vi "readAnPinVal.vi"(3 "YLDRMErrorInp":errorcluster, 4 "pin":u8, 5 "YLDRMPortInp":refnum<visa-resource-name>) -> (0 "YLDRMErrorOut":errorcluster, 1 "out":u16, 2 "YLDRMPortOut":refnum<visa-resource-name>)   [LabVIEW 2015]
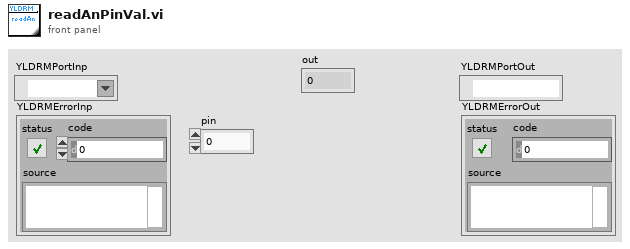
[diagram p1: front panel]
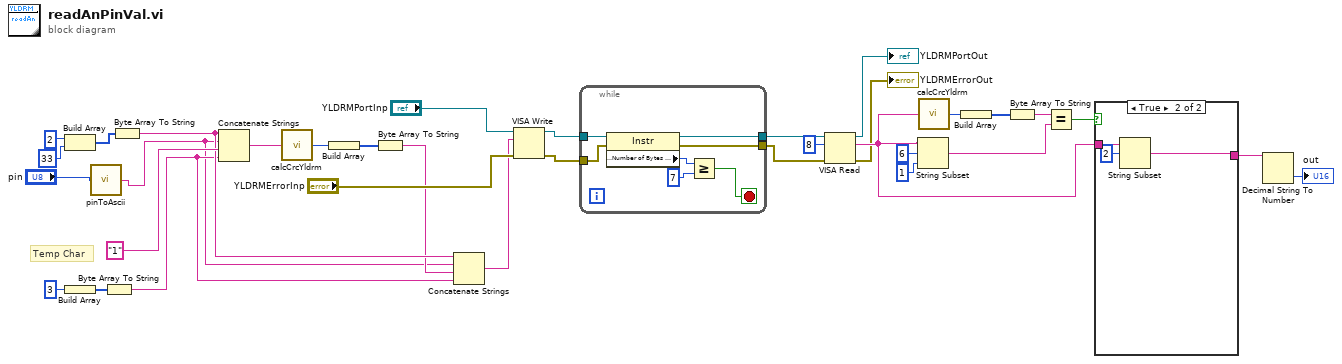
[diagram p0: block diagram]
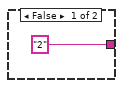
[diagram p2: hidden frame]
diagram:
  # "Temp Char"
  n1 = Build Array(2, 33) -> (w32:i32[])
  n2 = Build Array(3) -> (w30:i32[])
  n3 = call "pinToAscii.vi"("inp"="pin") -> ("out"=w1:string)
  n4 = Byte Array To String(unsigned byte array=w30) -> (string=w6:string)
  n5 = Byte Array To String(unsigned byte array=w32) -> (string=w8:string)
  n6 = Concatenate Strings(w8, w1, "1", w6) -> (w27:string)
  n7 = call "calcCrcYldrm.vi"("inpStr"=w27) -> ("crcVal"=w29:u8)
  n8 = Build Array(w29) -> (w28:u8[])
  n9 = Byte Array To String(unsigned byte array=w28) -> (string=w7:string)
  n10 = Concatenate Strings(w8, w1, w7, w6) -> (w5:string)
  n11 = VISA Write(VISA resource name="YLDRMPortInp", write buffer=w5, error in (no error)="YLDRMErrorInp") -> (VISA resource name out=w23:refnum<visa-resource-name>, error out=w22:errorcluster)  [unwired: 1 out]
  n12 = while {
    tunnel: w23 -> [w41]
    tunnel: w22 -> [w40]
    tunnel: [w39] -> w21
    tunnel: [w38] -> w20
    stop <- w35 stop-if-true
    n13 = property class="Instr"(reference=w41, error in=w40) -> (reference out=w39:refnum<visa-resource-name>, error out=w38:errorcluster, "Serial Settings:Number of Bytes at Serial Port"=w37:u32)
    n14 = Greater Or Equal?(x=w37, y=u32 7) -> (x >= y?=w35:bool)
  }
  n15 = VISA Read(VISA resource name=w21, byte count=u32 8, error in (no error)=w20) -> (VISA resource name out=→"YLDRMPortOut":refnum<visa-resource-name>, read buffer=w11:string, error out=→"YLDRMErrorOut":errorcluster)  [unwired: 1 out]
  n16 = String Subset(string=w11, offset (0)=6, length (rest)=1 ("length (rest)")) -> (substring=w13:string)
  n17 = call "calcCrcYldrm.vi"("inpStr"=w11) -> ("crcVal"=w17:u8)
  n18 = Build Array(w17) -> (w18:u8[])
  n19 = Byte Array To String(unsigned byte array=w18) -> (string=w14:string)
  n20 = Equal?(x=w14, y=w13) -> (x = y?=w12:bool)
  n21 = case shown="True" w12 {
    tunnel: w11 -> [_ w45]
    tunnel: ["2" w43] -> w4
    frame False {
    }
    frame True {
      n22 = String Subset(string=w45, offset (0)=2) -> (substring=w43:string)  [unwired: 1 in]
    }
  }
  n23 = Decimal String To Number(string=w4) -> (number=→"out":i32)  [unwired: 2 in, 1 out]
